vi "C37 Scale Analog Signals.vi"(7 "Analog Scaling":T1, 11 "Analog Values":sgl[](array[numeric])) -> (3 "Scaled Analog Values":sgl[](array[numeric]))   [LabVIEW 2013, in "C37118-DLL.lvlib"]
uses:
  C37118-DLL.lvlib
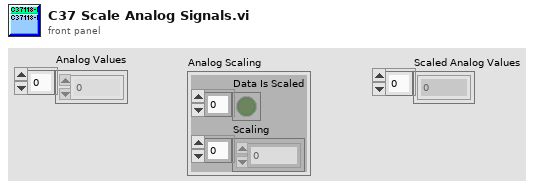
[diagram p1: front panel]
types:
  T1 = cluster{"Data Is Scaled":bool[], "Scaling":sgl[]}
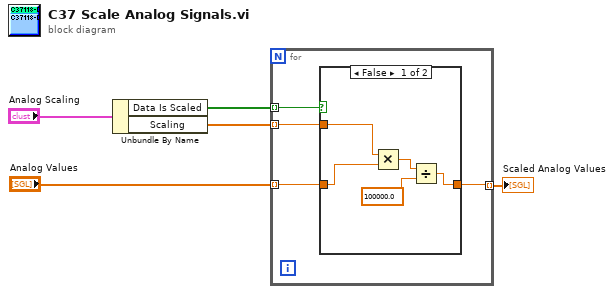
[diagram p0: block diagram]
diagram:
  n1 = Unbundle By Name("Analog Scaling") -> ("Data Is Scaled"=w4:bool[], "Scaling"=w3:sgl[])
  n2 = for {
    tunnel: w4 -> [w9] mode=indexing
    tunnel: w3 -> [w8] mode=indexing
    tunnel: "Analog Values" -> [w7] mode=indexing
    tunnel: [w6] -> w1 mode=indexing
    n3 = case shown="False" w9 {
      tunnel: w8 -> [w14 _]
      tunnel: w7 -> [w13 w15]
      tunnel: [w12 w15] -> w6
      frame False {
        n4 = Multiply(x=w14, y=w13) -> (x*y=w11:sgl)
        n5 = Divide(x=w11, y=sgl 100000.0) -> (x/y=w12:sgl)
      }
      frame True {
      }
    }
  }
  "Scaled Analog Values" <- w1
